vi "PathPlanner_PathFinding_SetStartingPosition.vi"(11 "StartPosition":T1 {"Y" format="%14.3f"; "X" format="%14.3f"}) -> ()   [LabVIEW 2019, in "PathPlanner24.lvlib"]
uses:
  PathPlanner24.lvlib
  <vilib>/Rock Robotics/WPI/ThirdParty/JAS_Junk/TrajLib/TypeDef/TRANSLATION2D.ctl
  ENum/PathPlanner_PathFinding_Cmd_ENUM.ctl
  <vilib>/Rock Robotics/WPI/ThirdParty/JAS_Junk/TrajLib/Translation2d_GetXY.vi
  PathPlanner_GridPosition_New.vi
  PathPlanner_PathFinder_GetAllNeighbors.vi
  PathPlanner_GridPosition_Get.vi
  PathPlanner_PathFinder_Globals.vi
  <vilib>/Rock Robotics/WPI/ThirdParty/JAS_Junk/TrajLib/Trajectory_Library.lvlib
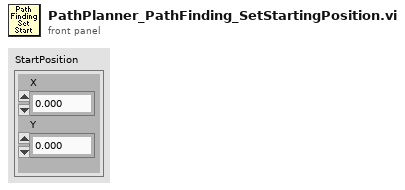
[diagram p1: front panel]
types:
  T1 = typedef "Trajectory_Library.lvlib/TRANSLATION2D.ctl" = cluster{"X":dbl, "Y":dbl}
  T2 = typedef "PathPlanner24.lvlib/PathPlannerFinderGridPosition.ctl" = cluster{"X":i32, "Y":i32}
  T3 = typedef "PathPlanner24.lvlib/PathPlanner_PathFinding_Cmd_ENUM.ctl" = enum16{"Do Nothing", "Reset", "Minor", "Reset and Minor", "Major", "Reset and Major", "Minor and Major", "Reset, Minor, Major"}
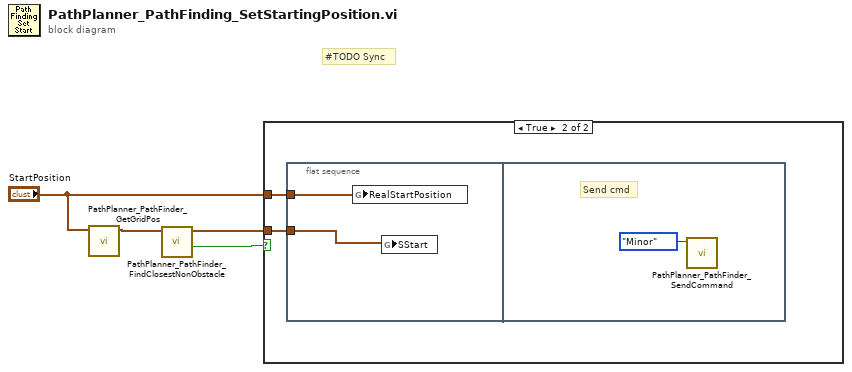
[diagram p0: block diagram]
diagram:
  # "#TODO Sync"
  n1 = call "PathPlanner_PathFinder_GetGridPos.vi"("RealGridPos"="StartPosition") -> ("GridPosition"=w4:T2)  [unwired: 10 in]
  n2 = call "PathPlanner_PathFinder_FindClosestNonObstacle.vi"("GridPosition"=w4) -> ("Found"=w3:bool, "NonObstacleGridPositin"=w2:T2)  [unwired: 9 in]
  n3 = case shown="True" w3 {
    tunnel: w2 -> [_ w6]
    tunnel: "StartPosition" -> [_ w5]
    frame False {
      # "Not found\nleave alone"
    }
    frame True {
      n4 = flat-sequence {
        tunnel: w6 -> [w8]
        tunnel: w5 -> [w7]
        frame #0 {
          n5 = global write "PathPlanner_PathFinder_Globals.vi" "RealStartPosition"(w7) -> ()
          n6 = global write "PathPlanner_PathFinder_Globals.vi" "SStart"(w8) -> ()
        }
        frame #1 {
          # "Send cmd"
          n7 = call "PathPlanner_PathFinder_SendCommand.vi"("PathFindingCommand"=PathPlanner_PathFinding_Cmd_ENUM."Minor") -> ()  [unwired: 10 in, 1 out]
        }
      }
    }
  }
